vi "Ex5_Reservoir.vi"() -> ()   [LabVIEW 2018]
panel:
  in  "Débit":u8(slide)=1 min=1 max=10 scale=1.0..10.0
  out "Réservoir":u16(slide) scale=0.0..1000.0
  in  "Consigne":u16(slide) max=1000 scale=0.0..1000.0
  in  "stop":bool
  # "[L/s]"
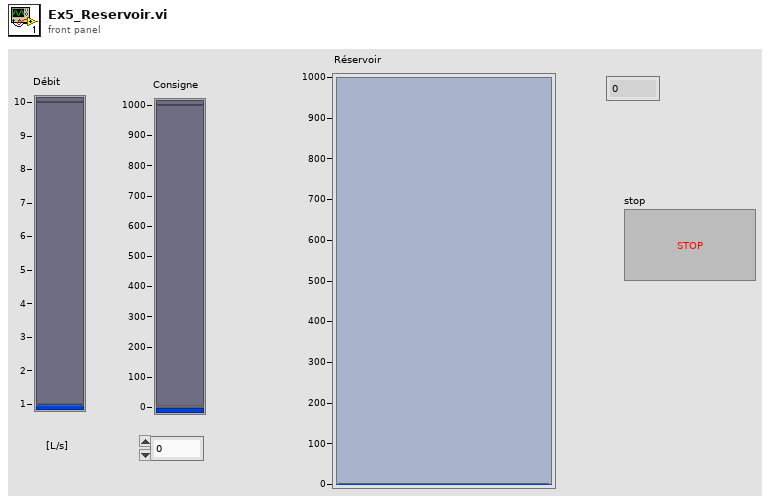
[diagram p1: front panel]
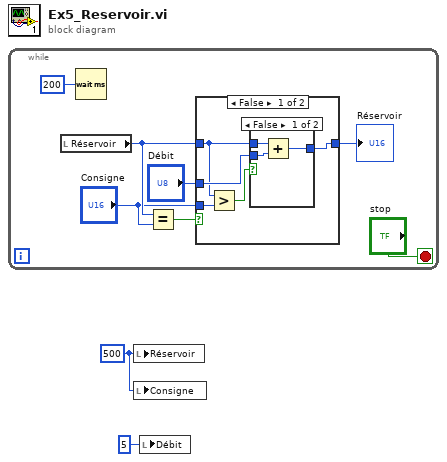
[diagram p0: block diagram]
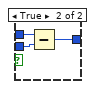
[diagram p2: hidden frame]
diagram:
  w2 = u16 500 ("Réservoir")
  n1 = while {
    stop <- "stop" stop-if-true
    n2 = local read "Réservoir"() -> (w5:u16)
    n3 = Wait (ms)(milliseconds to wait=u32 200) -> ()  [unwired: 1 out]
    n4 = Equal?(x=w5, y="Consigne") -> (x = y?=w4:bool)
    n5 = case shown="False" w4 {
      tunnel: w5 -> [w11 w21]
      tunnel: [w12 w21] -> w6
      tunnel: "Débit" -> [w13 _]
      tunnel: "Consigne" -> [w10 _]
      frame False {
        n6 = Greater?(x=w11, y=w10) -> (0:w14:bool)
        n7 = case shown="False" w14 {
          tunnel: w11 -> [w17 w20]
          tunnel: w13 -> [w16 w19]
          tunnel: [w15 w18] -> w12
          frame False {
            n8 = Add(x=w17, y=w16) -> (x+y=w15:u16)
          }
          frame True {
            n9 = Subtract(x=w20, y=w19) -> (x-y=w18:u16)
          }
        }
      }
      frame True {
      }
    }
    "Réservoir" <- w6
  }
  n10 = local write "Réservoir"(w2) -> ()
  n11 = local write "Consigne"(w2) -> ()
  n12 = local write "Débit"(u8 5 ("Débit")) -> ()
